vi "Measurement UI.vi"() -> ()   [LabVIEW 2021, in "Multi-Channel Output Voltage Accuracy_PMIC.lvlib"]
uses:
  Multi-Channel Output Voltage Accuracy_PMIC.lvlib
panel:
  in  "MeasGraphs":T1(tab)
  out "LoadVoltageGraph":waveform(dbl)[](graph) caption="AC"
  out "Maximum output voltage(V)":dbl[](array[numeric])
  out "Minimum output voltage(V)":dbl[](array[numeric])
  out "Average output voltage accuracy(V)":dbl[](array[numeric])
  out "Average output voltage deviation(%)":dbl[](array[numeric])
  out "Average measured output voltages(V)":dbl[](array[numeric])
  out "Output channel alias":string[](array[string])
  in  "Output channel alias":string[](array[string])
  in  "Load voltage limit ranges":dbl[](array[numeric])
  out "Load voltages":dbl[](array[numeric])
  in  "Nominal output voltages":dbl[](array[numeric])
  in  "Load current levels":dbl[](array[numeric])
  in  "Load resource names":string[](array[string])
  in  "Source resource name":string caption="RESOURCE NAME"
  out "dt":dbl[](array[numeric])
  out "MeasTable":string[][](table)
  out "Status":string
  in  "Load configuration parameters":T2(array[cluster]) {"Nominal output voltage" format="%#_6pV"; "Load voltage limit range" format="%#_6pV"; "Load current level" format="%#_6pA"}
  in  "PPSResourceName":refnum<k15> caption="RESOURCE NAME"
  in  "DUT setup time":dbl=1.0 caption="DUT SETUP TIME" format="%#_6ps"
  in  "Measurement time":dbl=0.005 caption="MEASUREMENT TIME" format="%#_6ps"
  in  "Aperture time":dbl=0.005 caption="APERTURE TIME" format="%#_6ps"
  in  "Source voltage level":dbl=6.0 caption="VOLTAGE LEVEL" format="%#_6pV"
  in  "Source current limit":dbl=25.0 caption="CURRENT LIMIT" format="%#_6pA"
  in  "Load configuration":string="Load configuration"
  in  "Source configuration":string="Source configuration"
  in  "Measurement settings":string="Measurement settings"
  in  "Mode of operation":T3(ring)=enum."Perform measurement" caption="MODE OF OPERATION"
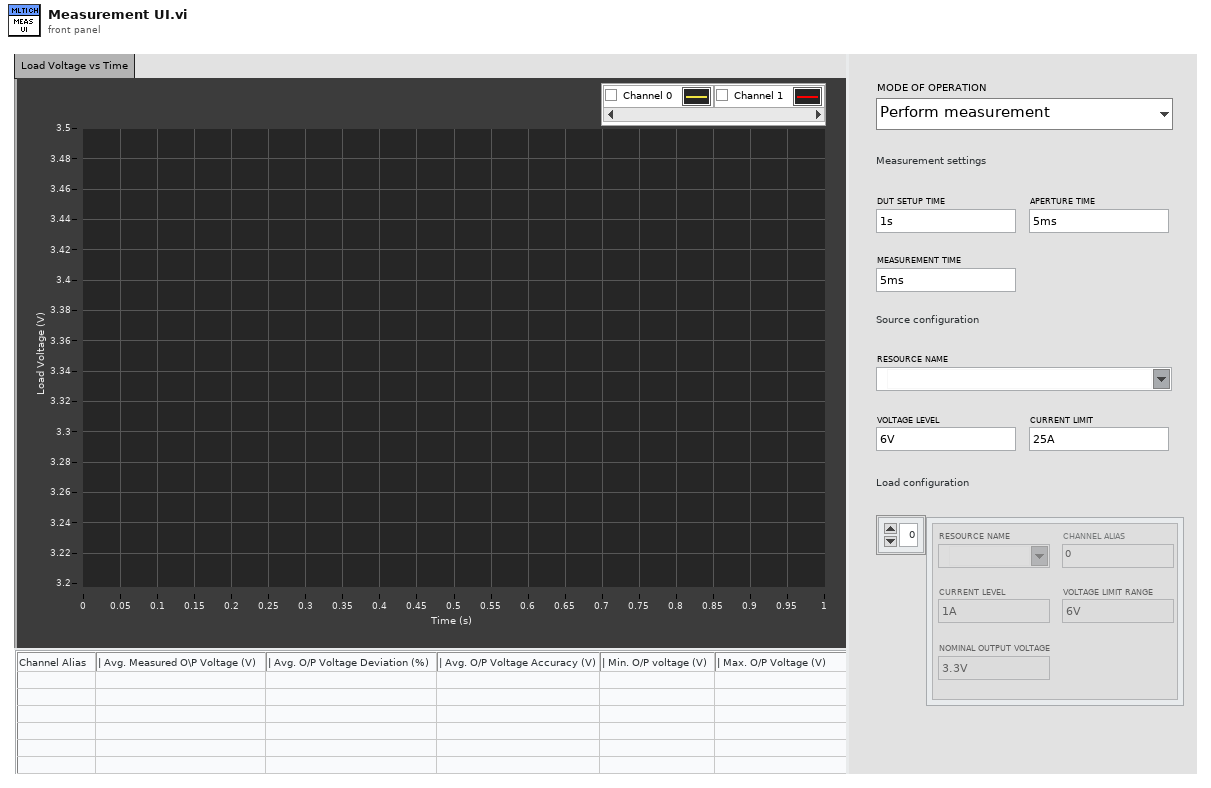
[diagram p1: front panel]
types:
  T1 = enum32{"Load Voltage vs Time", "Hidden Controls"}
  T2 = cluster{"ELOADResourceName":refnum<k15>, "Load current level":dbl, "Load voltage limit range":dbl, "Input channel":string, "Nominal output voltage":dbl}[]
  T3 = enum32{"Power on the DUT", "Perform measurement", "Power off the DUT"}
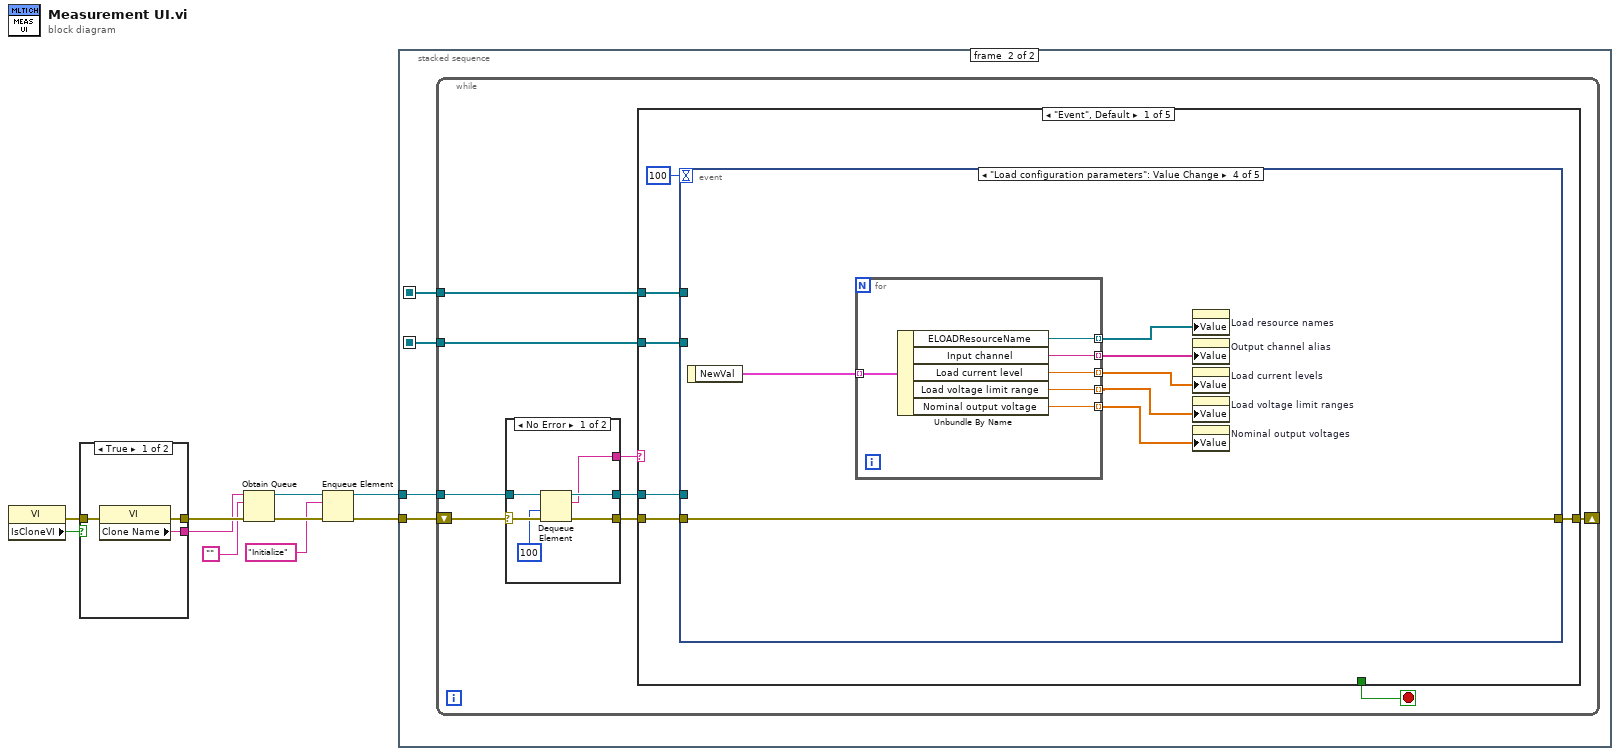
[diagram p0: block diagram]
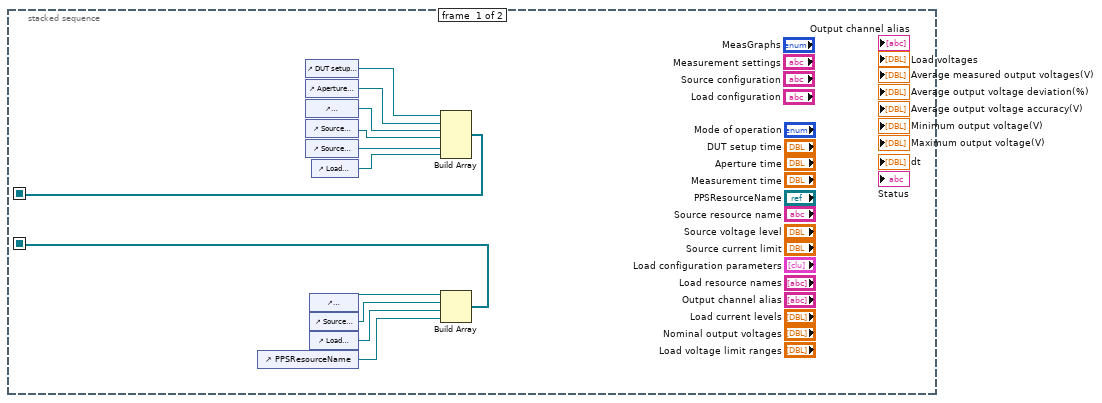
[diagram p2: hidden frame]
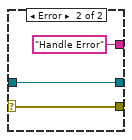
[diagram p3: hidden frame]
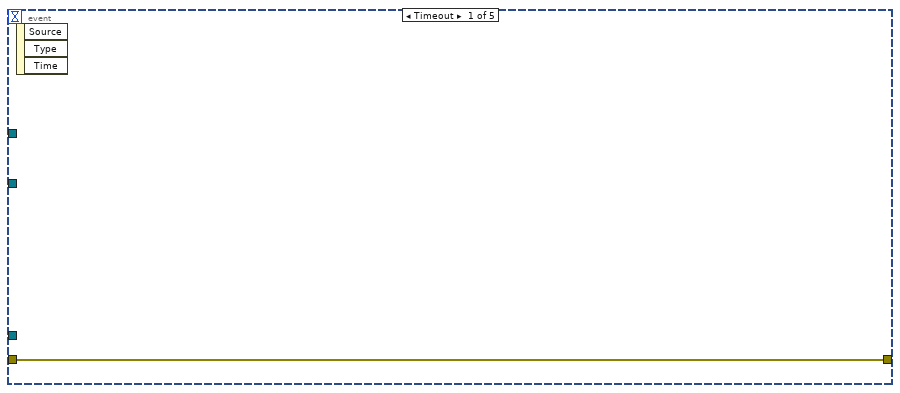
[diagram p4: hidden frame]
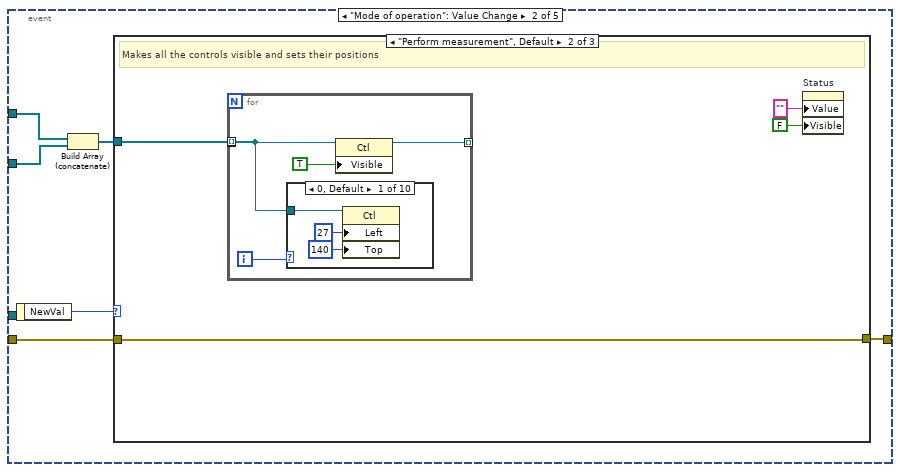
[diagram p5: hidden frame]
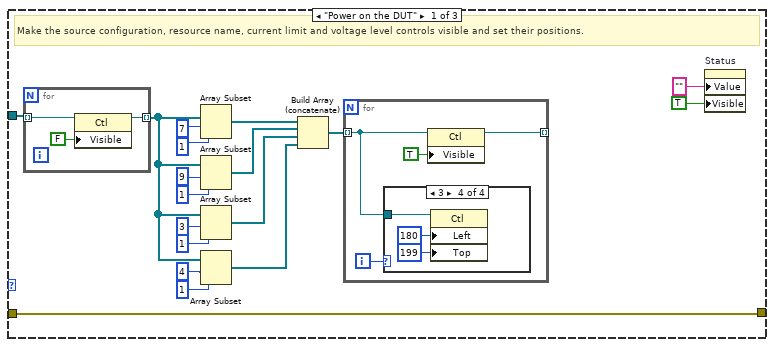
[diagram p6: hidden frame]
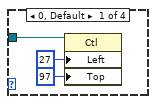
[diagram p7: hidden frame]
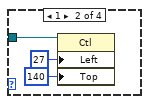
[diagram p8: hidden frame]
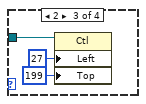
[diagram p9: hidden frame]
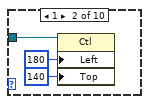
[diagram p10: hidden frame]
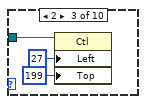
[diagram p11: hidden frame]
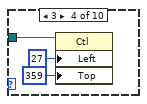
[diagram p12: hidden frame]
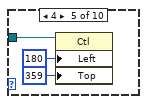
[diagram p13: hidden frame]
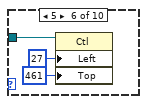
[diagram p14: hidden frame]
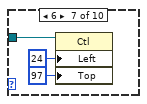
[diagram p15: hidden frame]
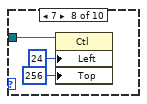
[diagram p16: hidden frame]
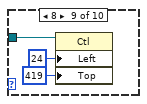
[diagram p17: hidden frame]
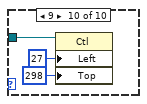
[diagram p18: hidden frame]
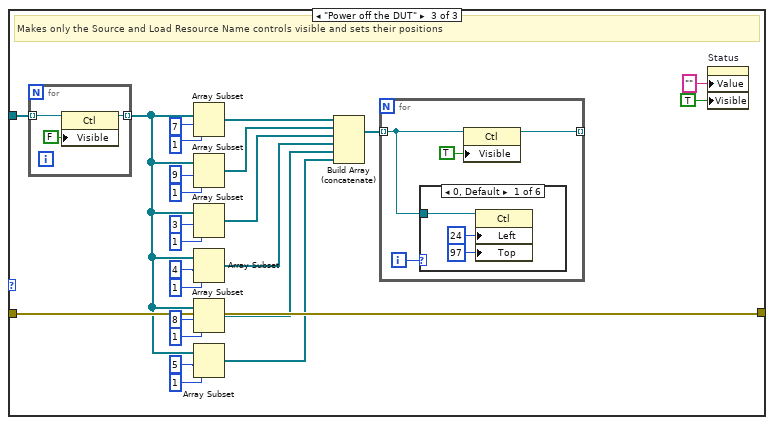
[diagram p19: hidden frame]
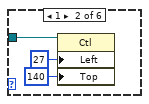
[diagram p20: hidden frame]
diagram:
  n1 = property class="VI"() -> (error out=w1:errorcluster, "IsCloneVI"=w2:bool)  [unwired: 2 in, 1 out]
  n2 = case shown="True" w2 {
    tunnel: [w13 w16] -> w10
    tunnel: [w12 w15] -> w9
    tunnel: w1 -> [w11 w14]
    frame True {
      n3 = property class="VI"(error in=w11) -> (error out=w13:errorcluster, "Clone Name"=w12:string)  [unwired: 1 in, 1 out]
    }
    frame False {
      n4 = property class="VI"(error in=w14) -> (error out=w16:errorcluster, "Name"=w15:string)  [unwired: 1 in, 1 out]
    }
  }
  n5 = Obtain Queue(name (unnamed)=w9, element data type="", error in (no error)=w10) -> (queue out=w6:refnum<queue>, error out=w8:errorcluster)  [unwired: 2 in, 1 out]
  n6 = Enqueue Element(queue=w6, element="Initialize", error in (no error)=w8) -> (queue out=w5:refnum<queue>, error out=w7:errorcluster)  [unwired: 1 in, 1 out]
  n7 = stacked-sequence {
    seq-local: [w18 _] -> [_ w30]
    seq-local: [w17 _] -> [_ w29]
    tunnel: w7 -> [_ w32]
    tunnel: w5 -> [_ w31]
    frame #0 {
      n8 = control-ref of="PPSResourceName"() -> (w19:refnum<vi>)
      n9 = control-ref of="DUT setup time"() -> (w28:refnum<vi>)
      n10 = control-ref of="Aperture time"() -> (w27:refnum<vi>)
      n11 = control-ref of="Measurement time"() -> (w26:refnum<vi>)
      n12 = control-ref of="Source voltage level"() -> (w25:refnum<vi>)
      n13 = control-ref of="Source current limit"() -> (w24:refnum<vi>)
      n14 = control-ref of="Measurement settings"() -> (w22:refnum<vi>)
      n15 = control-ref of="Source configuration"() -> (w21:refnum<vi>)
      n16 = control-ref of="Load configuration"() -> (w20:refnum<vi>)
      n17 = control-ref of="Load configuration parameters"() -> (w23:refnum<vi>)
      n18 = Build Array(w28, w27, w26, w25, w24, w23) -> (w18:refnum<vi>[])
      n19 = Build Array(w22, w21, w20, w19) -> (w17:refnum<vi>[])
    }
    frame #1 {
      n20 = while {
        shift-right: [w36] -> _
        shift-left: w32 -> [w41]
        tunnel: w31 -> [w39]
        tunnel: w30 -> [w34]
        tunnel: w29 -> [w33]
        stop <- w35 stop-if-true
        n21 = case shown="No Error" w41 {
          selector: w41 -> [w47 w50]
          tunnel: [w46 w50] -> w40
          tunnel: w39 -> [w45 w49]
          tunnel: [w44 w49] -> w38
          tunnel: [w43 "Handle Error"] -> w37
          frame No Error {
            n22 = Dequeue Element(queue=w45, timeout in ms (-1)=100, error in (no error)=w47) -> (queue out=w44:refnum<queue>, element=w43:string, error out=w46:errorcluster)  [unwired: 1 out]
          }
          frame Error {
          }
        }
        n23 = case shown="\"Event\", Default" w37 {
          tunnel: w40 -> [w55 w208 w216 w257 w258]
          tunnel: w38 -> [w53 _ _ w255 _]
          tunnel: [w56 w208 w216 w252 w258] -> w36
          tunnel: [_ FALSE _ TRUE _] -> w35
          tunnel: w34 -> [w52 _ _ _ _]
          tunnel: w33 -> [w51 _ _ _ _]
          frame "Event", Default {
            n24 = event shown="[3] \"Load configuration parameters\": Value Change" {
              selector: _ -> [_ _ _ _ _]
              dyn-events: _ -> [_ _ _ _ _]
              timeout: 100 -> [_ _ _ _ _]
              tunnel: [w57 w58 _ w189 w204] -> w56
              tunnel: w55 -> [w57 w59 _ w189 w205]
              tunnel: w53 -> [_ _ _ _ w203]
              tunnel: w52 -> [_ w62 _ _ _]
              tunnel: w51 -> [_ w61 _ _ _]
              event Timeout {
                n25 = event-data() -> ()  [unwired: 1 in, 3 out]
              }
              event "Mode of operation": Value Change {
                n26 = event-data() -> ("NewVal"=w63:T3)  [unwired: 1 in]
                n27 = Build Array (concatenate)(w62, w61) -> (w60:refnum<vi>[])
                n28 = case shown="\"Perform measurement\", Default" w63 {
                  tunnel: w60 -> [w73 w102 w146]
                  tunnel: w59 -> [w64 w101 w160]
                  tunnel: [w64 w101 w160] -> w58
                  frame "Power on the DUT" {
                    # "Make the source configuration, resource name, current limit and voltage level controls visible and set their positions."
                    n29 = for {
                      tunnel: w73 -> [w84] mode=indexing
                      tunnel: [w82] -> w70 mode=indexing
                      n30 = property class="Ctl"(reference=w84, "Visible"=FALSE) -> (reference out=w82:refnum<vi>)  [unwired: 1 in, 1 out]
                    }
                    n31 = Array Subset(array=w70, index=7 ("length"), length=1 ("index")) -> (w72:refnum<vi>[])
                    n32 = Array Subset(array=w70, index=9 ("length"), length=1 ("index")) -> (w71:refnum<vi>[])
                    n33 = Array Subset(array=w70, index=3 ("length"), length=1 ("index")) -> (w69:refnum<vi>[])
                    n34 = Array Subset(array=w70, index=4 ("length"), length=1 ("index")) -> (w67:refnum<vi>[])
                    n35 = Build Array (concatenate)(w72, w71, w69, w67) -> (w68:refnum<vi>[])
                    n36 = for {
                      tunnel: [w87] -> _ mode=indexing
                      tunnel: w68 -> [w85] mode=indexing
                      i -> [w86]
                      n37 = case shown="3" w86 {
                        tunnel: w85 -> [w91 w94 w97 w100]
                        frame 0, Default {
                          n38 = property class="Ctl"(reference=w91, "Left"=27 ("Position:Left"), "Top"=97 ("Position:Top")) -> ()  [unwired: 1 in, 2 out]
                        }
                        frame 1 {
                          n39 = property class="Ctl"(reference=w94, "Left"=27 ("Position:Left"), "Top"=140 ("Position:Top")) -> ()  [unwired: 1 in, 2 out]
                        }
                        frame 2 {
                          n40 = property class="Ctl"(reference=w97, "Left"=27 ("Position:Left"), "Top"=199 ("Position:Top")) -> ()  [unwired: 1 in, 2 out]
                        }
                        frame 3 {
                          n41 = property class="Ctl"(reference=w100, "Left"=180 ("Position:Left"), "Top"=199 ("Position:Top")) -> ()  [unwired: 1 in, 2 out]
                        }
                      }
                      n42 = property class="Ctl"(reference=w85, "Visible"=TRUE) -> (reference out=w87:refnum<vi>)  [unwired: 1 in, 1 out]
                    }
                    n43 = property on="Status" class="Str"("Value"="" ("Status"), "Visible"=TRUE) -> ()  [unwired: 2 in, 2 out]
                  }
                  frame "Perform measurement", Default {
                    # "Makes all the controls visible and sets their positions"
                    n44 = for {
                      tunnel: [w105] -> _ mode=indexing
                      tunnel: [w107] -> _ mode=indexing
                      tunnel: w102 -> [w105] mode=indexing
                      i -> [w106]
                      n45 = case shown="0, Default" w106 {
                        tunnel: w105 -> [w111 w114 w117 w120 w123 w126 w129 w132 w135 w138]
                        frame 0, Default {
                          n46 = property class="Ctl"(reference=w111, "Left"=27 ("Position:Left"), "Top"=140 ("Position:Top")) -> ()  [unwired: 1 in, 2 out]
                        }
                        frame 1 {
                          n47 = property class="Ctl"(reference=w114, "Left"=180 ("Position:Left"), "Top"=140 ("Position:Top")) -> ()  [unwired: 1 in, 2 out]
                        }
                        frame 2 {
                          n48 = property class="Ctl"(reference=w117, "Left"=27 ("Position:Left"), "Top"=199 ("Position:Top")) -> ()  [unwired: 1 in, 2 out]
                        }
                        frame 3 {
                          n49 = property class="Ctl"(reference=w120, "Left"=27 ("Position:Left"), "Top"=359 ("Position:Top")) -> ()  [unwired: 1 in, 2 out]
                        }
                        frame 4 {
                          n50 = property class="Ctl"(reference=w123, "Left"=180 ("Position:Left"), "Top"=359 ("Position:Top")) -> ()  [unwired: 1 in, 2 out]
                        }
                        frame 5 {
                          n51 = property class="Ctl"(reference=w126, "Left"=27 ("Position:Left"), "Top"=461 ("Position:Top")) -> ()  [unwired: 1 in, 2 out]
                        }
                        frame 6 {
                          n52 = property class="Ctl"(reference=w129, "Left"=24 ("Position:Left"), "Top"=97 ("Position:Top")) -> ()  [unwired: 1 in, 2 out]
                        }
                        frame 7 {
                          n53 = property class="Ctl"(reference=w132, "Left"=24 ("Position:Left"), "Top"=256 ("Position:Top")) -> ()  [unwired: 1 in, 2 out]
                        }
                        frame 8 {
                          n54 = property class="Ctl"(reference=w135, "Left"=24 ("Position:Left"), "Top"=419 ("Position:Top")) -> ()  [unwired: 1 in, 2 out]
                        }
                        frame 9 {
                          n55 = property class="Ctl"(reference=w138, "Left"=27 ("Position:Left"), "Top"=298 ("Position:Top")) -> ()  [unwired: 1 in, 2 out]
                        }
                      }
                      n56 = property class="Ctl"(reference=w105, "Visible"=TRUE) -> (reference out=w107:refnum<vi>)  [unwired: 1 in, 1 out]
                    }
                    n57 = property on="Status" class="Str"("Value"="" ("Status"), "Visible"=FALSE) -> ()  [unwired: 2 in, 2 out]
                  }
                  frame "Power off the DUT" {
                    # "Makes only the Source and Load Resource Name controls visible and sets their positions"
                    n58 = for {
                      tunnel: w146 -> [w164] mode=indexing
                      tunnel: [w163] -> w141 mode=indexing
                      n59 = property class="Ctl"(reference=w164, "Visible"=FALSE) -> (reference out=w163:refnum<vi>)  [unwired: 1 in, 1 out]
                    }
                    n60 = Array Subset(array=w141, index=7 ("length"), length=1 ("index")) -> (w151:refnum<vi>[])
                    n61 = Array Subset(array=w141, index=9 ("length"), length=1 ("index")) -> (w150:refnum<vi>[])
                    n62 = Array Subset(array=w141, index=3 ("length"), length=1 ("index")) -> (w149:refnum<vi>[])
                    n63 = Array Subset(array=w141, index=4 ("length"), length=1 ("index")) -> (w147:refnum<vi>[])
                    n64 = Array Subset(array=w141, index=8 ("length"), length=1 ("index")) -> (w140:refnum<vi>[])
                    n65 = Array Subset(array=w141, index=5 ("length"), length=1 ("index")) -> (w139:refnum<vi>[])
                    n66 = Build Array (concatenate)(w151, w150, w149, w147, w140, w139) -> (w148:refnum<vi>[])
                    n67 = for {
                      tunnel: [w168] -> _ mode=indexing
                      tunnel: w148 -> [w166] mode=indexing
                      i -> [w167]
                      n68 = case shown="0, Default" w167 {
                        tunnel: w166 -> [w172 w175 w178 w181 w182 w185]
                        frame 0, Default {
                          n69 = property class="Ctl"(reference=w172, "Left"=24 ("Position:Left"), "Top"=97 ("Position:Top")) -> ()  [unwired: 1 in, 2 out]
                        }
                        frame 1 {
                          n70 = property class="Ctl"(reference=w175, "Left"=27 ("Position:Left"), "Top"=140 ("Position:Top")) -> ()  [unwired: 1 in, 2 out]
                        }
                        frame 2 {
                          n71 = property class="Ctl"(reference=w178, "Left"=27 ("Position:Left"), "Top"=199 ("Position:Top")) -> ()  [unwired: 1 in, 2 out]
                        }
                        frame 3 {
                          n72 = property class="Ctl"(reference=w181, "Left"=180 ("Position:Left"), "Top"=199 ("Position:Top")) -> ()  [unwired: 1 in, 2 out]
                        }
                        frame 4 {
                          n73 = property class="Ctl"(reference=w182, "Left"=27 ("Position:Left"), "Top"=254 ("Position:Top")) -> ()  [unwired: 1 in, 2 out]
                        }
                        frame 5 {
                          n74 = property class="Ctl"(reference=w185, "Left"=27 ("Position:Left"), "Top"=303 ("Position:Top")) -> ()  [unwired: 1 in, 2 out]
                        }
                      }
                      n75 = property class="Ctl"(reference=w166, "Visible"=TRUE) -> (reference out=w168:refnum<vi>)  [unwired: 1 in, 1 out]
                    }
                    n76 = property on="Status" class="Str"("Value"="" ("Status"), "Visible"=TRUE) -> ()  [unwired: 2 in, 2 out]
                  }
                }
              }
              event "PPSResourceName": Value Change {
                n77 = event-data() -> ("NewVal"=w188:refnum<k15>)  [unwired: 1 in]
                n78 = property on="Source resource name" class="Str"("Value"=w188) -> ()  [unwired: 2 in, 2 out]
              }
              event "Load configuration parameters": Value Change {
                n79 = event-data() -> ("NewVal"=w195:T2)  [unwired: 1 in]
                n80 = for {
                  tunnel: w195 -> [w201] mode=indexing
                  tunnel: [w200] -> w194 mode=indexing
                  tunnel: [w199] -> w193 mode=indexing
                  tunnel: [w198] -> w190 mode=indexing
                  tunnel: [w197] -> w192 mode=indexing
                  tunnel: [w196] -> w191 mode=indexing
                  n81 = Unbundle By Name(w201) -> ("ELOADResourceName"=w200:refnum<k15>, "Input channel"=w199:string, "Load current level"=w198:dbl, "Load voltage limit range"=w197:dbl, "Nominal output voltage"=w196:dbl)
                }
                n82 = property on="Load resource names" class="Arr (strict)"("Value"=w194) -> ()  [unwired: 2 in, 2 out]
                n83 = property on="Output channel alias" class="Arr (strict)"("Value"=w193) -> ()  [unwired: 2 in, 2 out]
                n84 = property on="Load current levels" class="Arr (strict)"("Value"=w190) -> ()  [unwired: 2 in, 2 out]
                n85 = property on="Load voltage limit ranges" class="Arr (strict)"("Value"=w192) -> ()  [unwired: 2 in, 2 out]
                n86 = property on="Nominal output voltages" class="Arr (strict)"("Value"=w191) -> ()  [unwired: 2 in, 2 out]
              }
              event Panel Close? {
                n87 = event-data() -> ()  [unwired: 1 in, 4 out]
                n88 = Enqueue Element(queue=w203, element="Exit", error in (no error)=w205) -> (error out=w204:errorcluster)  [unwired: 1 in, 2 out]
                n89 = event-data("Discard?"=TRUE) -> ()  [unwired: 1 in, 1 out]
              }
            }
          }
          frame "Initialize" {
          }
          frame "Post UI Update" {
            # "This case will be triggered, after framework updates the User interface with result values."
            n90 = local read "Output channel alias"() -> (w214:string[])
            n91 = local read "Average measured output voltages(V)"() -> (w217:dbl[])
            n92 = local read "Average output voltage deviation(%)"() -> (w215:dbl[])
            n93 = local read "Average output voltage accuracy(V)"() -> (w211:dbl[])
            n94 = local read "Load voltages"() -> (w222:dbl[])
            n95 = local read "Maximum output voltage(V)"() -> (w210:dbl[])
            n96 = local read "Minimum output voltage(V)"() -> (w212:dbl[])
            n97 = for {
              tunnel: w214 -> [w225] mode=indexing
              tunnel: [w225] -> w213 mode=indexing
              i -> [w224]
              n98 = property on="LoadVoltageGraph" class="WFGraph (strict)"("Active Plot"=w224, "Plot.Plot Name"=w225) -> ()  [unwired: 2 in, 2 out]
            }
            n99 = local read "dt"() -> (w219:dbl[])
            n100 = Array Size(array=w222) -> (size(s)=w221:i32)
            n101 = Array Size(array=w219) -> (size(s)=w209:i32)
            n102 = Divide(x=w221, y=w209) -> (x/y=w220:dbl)
            n103 = for {
              N: w209 -> [_]
              tunnel: [w250] -> w223 mode=indexing
              tunnel: w220 -> [w248]
              shift-right: [w246] -> _
              shift-left: w222 -> [w249]
              tunnel: w219 -> [w244] mode=indexing
              n104 = Delete From Array(array=w249, length=w248, index=0) -> (deleted portion=w247:dbl[], array with subset deleted=w246:dbl[])
              n105 = Bundle By Name("dt"=w244, "Y"=w247) -> (w250:waveform(dbl))  [unwired: 1 in]
            }
            "LoadVoltageGraph" <- w223
            n106 = for {
              N: w209 -> [_]
              tunnel: w211 -> [w233] mode=indexing
              tunnel: w217 -> [w235] mode=indexing
              tunnel: [w241] -> w218 mode=indexing
              tunnel: w213 -> [w240] mode=indexing
              tunnel: w215 -> [w234] mode=indexing
              tunnel: w212 -> [w232] mode=indexing
              tunnel: w210 -> [w231] mode=indexing
              w226 = "|" ("initial string")
              n107 = Format Into String(format string="%0.9f" ("initial string"), w235) -> (resulting string=w242:string)  [unwired: 2 in, 1 out]
              n108 = Format Into String(format string="%0.9f" ("initial string"), initial string=w226, w234) -> (resulting string=w230:string)  [unwired: 1 in, 1 out]
              n109 = Format Into String(format string="%0.9f" ("initial string"), initial string=w226, w233) -> (resulting string=w229:string)  [unwired: 1 in, 1 out]
              n110 = Format Into String(format string="%0.9f" ("initial string"), initial string=w226, w232) -> (resulting string=w228:string)  [unwired: 1 in, 1 out]
              n111 = Format Into String(format string="%0.9f" ("initial string"), initial string=w226, w231) -> (resulting string=w227:string)  [unwired: 1 in, 1 out]
              n112 = Build Array(w240, w242, w230, w229, w228, w227) -> (w241:string[])
            }
            "MeasTable" <- w218
          }
          frame "Exit" {
            # "This case is triggered to close the User Interface from framework"
            n113 = Flush Queue(queue=w255, error in (no error)=w257) -> (queue out=w254:refnum<queue>, error out=w253:errorcluster)  [unwired: 1 out]
            n114 = Release Queue(queue=w254, force destroy? (F)=TRUE, error in (no error)=w253) -> (error out=w252:errorcluster)  [unwired: 2 out]
          }
          frame "Handle Error" {
          }
        }
      }
    }
  }
